vi "_fgv_debug.vi"(7 "Operation":T1=enum."ReadCommand", 8 "error in":errorcluster caption="error in (no error)", 9 "Command in":string, 11 "VISA resource name":refnum<visa-resource-name>) -> (0 "error out":errorcluster, 3 "VISA resource name out":refnum<visa-resource-name>)   [LabVIEW 2020, in "Rohde&Schwarz RTx Oscilloscopes.lvlib" / "rsidr_core.lvlib"]
uses:
  rsidr_core.lvlib
  _type_Operation_Fgv_Debug.ctl
  type_Error_Codes.ctl
  Match Regular Expression.xnode
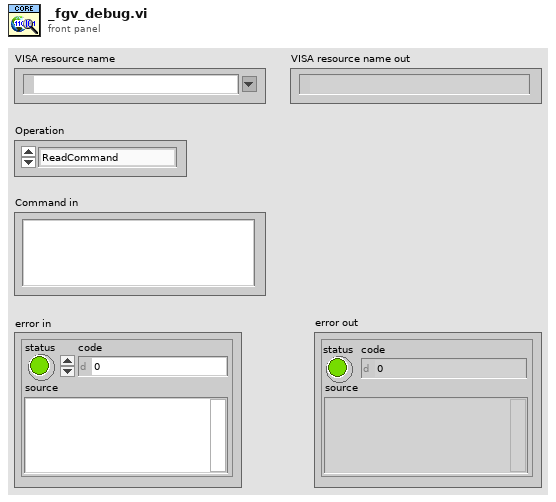
[diagram p1: front panel]
types:
  T1 = typedef "Rohde&Schwarz RTx Oscilloscopes.lvlib/rsidr_core.lvlib/_type_Operation_Fgv_Debug.ctl" = enum16{"Reset", "ReadCommand", "SetCommand"}
  T2 = typedef "Rohde&Schwarz RTx Oscilloscopes.lvlib/rsidr_core.lvlib/type_Error_Codes.ctl" = enum16{"No_error", "VISA_err_ResourceNotFound", "VISA_err_Timeout", "VISA_warn_MoreDataAvailable", "RS_err_MissingCallback", "RS_err_InvalidAttribute", "RS_err_InvalidValue", "RS_err_UnknownResource", "RS_err_AlreadyInitialized", "RS_err_InstrumentStatus", "RS_err_BadRepCapName", "RS_err_TypesMismatch", "RS_err_ValueNotSupported", "RS_err_InvalidRngTable", "RS_err_IDqueryFail", "RS_err_UnexpResponse", "VISA_warn_ConfigNotLoaded", "RS_err_AttributeNotReadable", "RS_err_AttributeNotWritable", "RS_err_InstrumentType", "RS_err_InstrumentOption", "VISA_err_InvalidSize", "RS_err_ReliabilityIndicator", "VISA_warn_UnknownStatus", "VISA_warn_TermCharRead", "VISA_err_IO_error", "RS_err_FunctionNotSupported", "VISA_warn_QueueEmpty"}
  T3 = typedef "Rohde&Schwarz RTx Oscilloscopes.lvlib/rsidr_core.lvlib/type_Session_Data.ctl" = cluster{"IDN string":string, "Instrument FW":string, "Instr type":string, "Instr type for err. msg.":string, "Installed Options":string[], "Ignore Error Messages":string, "Logging params":variant, "OPC Timeout":i32, "VISA Timeout":i32, "STB Poll VISA Timeout":i32, "Additional Flags":i32, "Wait Before Read":i32, "Wait Before Write":i32, "Option String Flags":i32, "IO Segment Size":i64, "VISA Access Mode":T4, "Interface Type":T5, "OPC Wait Mode":T6, "Bin Float Number  Format":T7, "Bin Integer Number Format":T8, "Simulate":bool, "VXIcapable":bool, "Duplicate Session":bool, "Add LF to Write":bool, "Logging":bool, "Fast Sweep":bool, "Query Instrument Status":bool, "Check Range":bool, "Check Options":bool, "OPC-sync Attr Writes":bool, "OPC-sync Attr Queries":bool}
  T4 = typedef "Rohde&Schwarz RTx Oscilloscopes.lvlib/rsidr_core.lvlib/type_VisaAccessMode.ctl" = u16
  T5 = typedef "Rohde&Schwarz RTx Oscilloscopes.lvlib/rsidr_core.lvlib/type_InterfaceType.ctl" = enum16{"Unknown", "GPIB", "VXI", "GPIB_VXI", "ASRL", "PXI", "TCPIP", "USB", "SOCKET"}
  T6 = typedef "Rohde&Schwarz RTx Oscilloscopes.lvlib/rsidr_core.lvlib/type_OPC_Wait_Mode.ctl" = enum16{"STBpolling", "STBpollingSlow", "STBpollingSuperSlow", "ServiceRequest", "OPCquery"}
  T7 = typedef "Rohde&Schwarz RTx Oscilloscopes.lvlib/rsidr_core.lvlib/type_Binary_Float_Number_Format.ctl" = enum16{"Float_4_Bytes_Swapped", "Float_4_Bytes", "Double_8_Bytes_Swapped", "Double_8_Bytes"}
  T8 = typedef "Rohde&Schwarz RTx Oscilloscopes.lvlib/rsidr_core.lvlib/type_Binary_Integer_Number_Format.ctl" = enum16{"Int32_4_Bytes_Swapped", "Int32_4 Bytes", "Int16_2_Bytes_Swapped", "Int16_2_Bytes"}
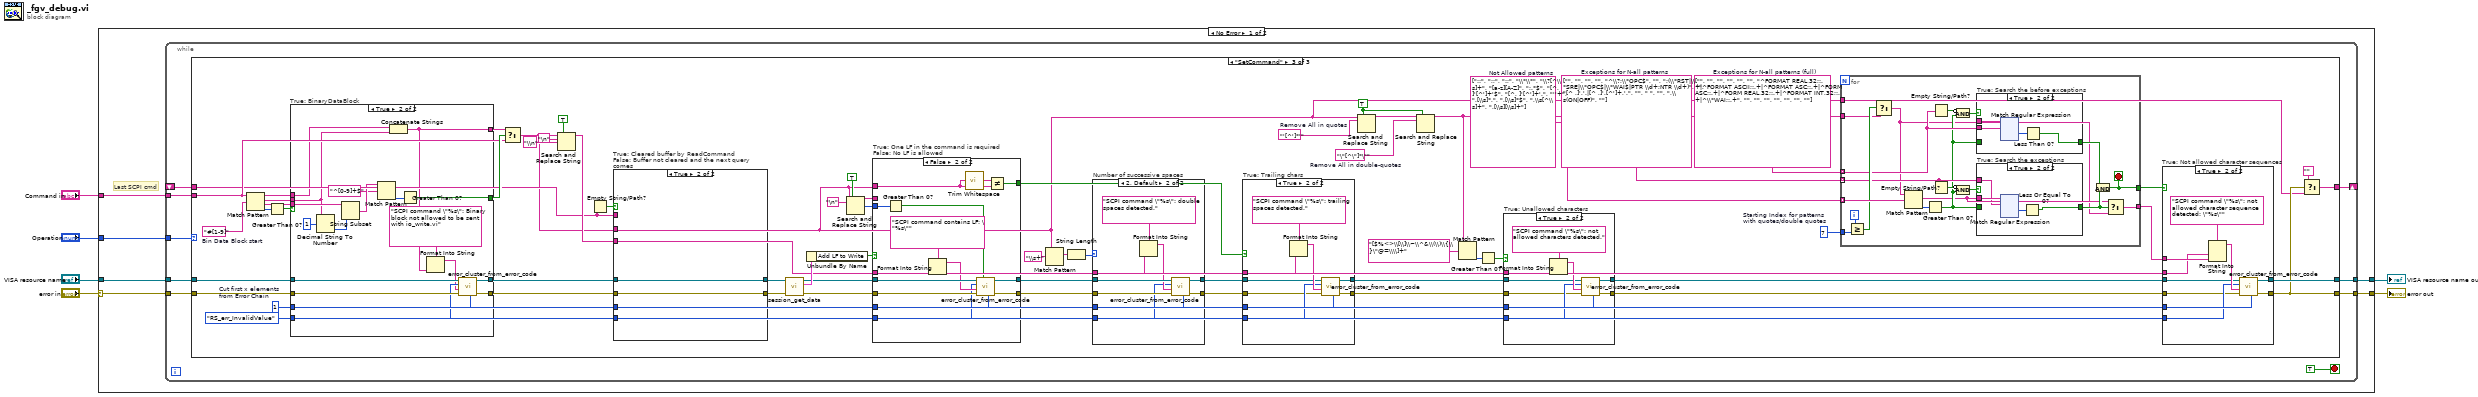
[diagram p0: block diagram]
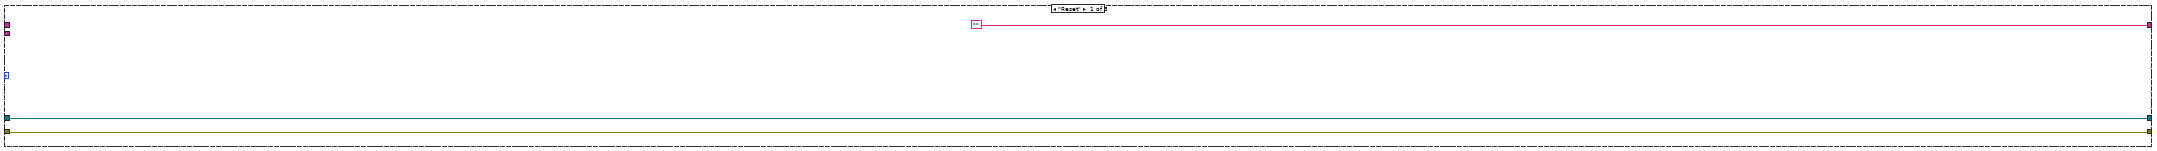
[diagram p2: hidden frame]
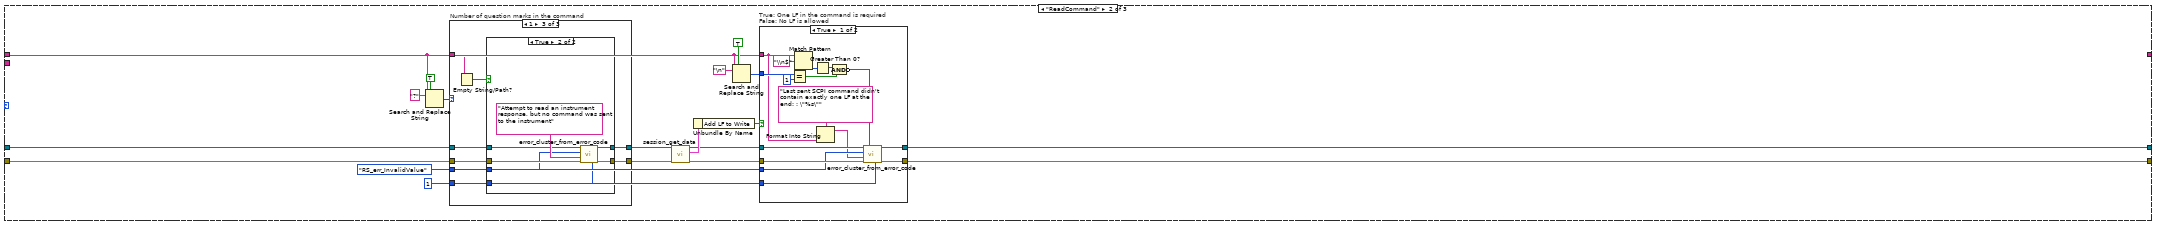
[diagram p3: hidden frame]
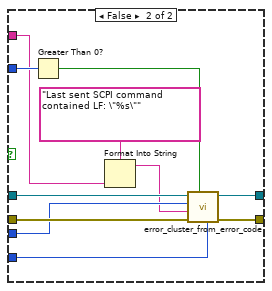
[diagram p4: hidden frame]
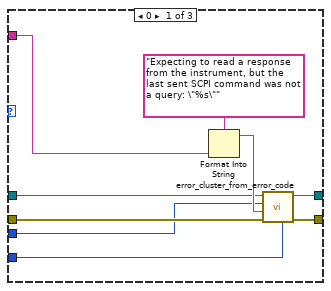
[diagram p5: hidden frame]
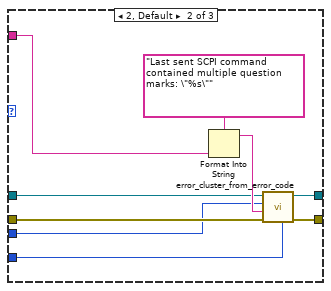
[diagram p6: hidden frame]
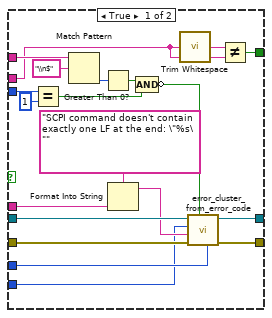
[diagram p14: hidden frame]
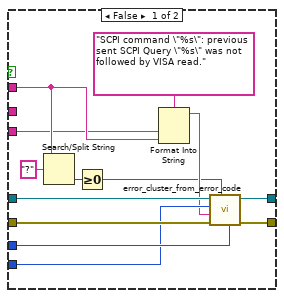
[diagram p16: hidden frame]
diagram:
  n1 = case shown="No Error" "error in" {
    selector: "error in" -> [w8 w536]
    tunnel: [w10 w536] -> w2
    tunnel: "Operation" -> [w12 _]
    tunnel: "Command in" -> [w11 _]
    tunnel: "VISA resource name" -> [w7 w535]
    tunnel: [w9 w535] -> w1
    frame No Error {
      # "Last SCPI cmd"
      n2 = while {
        shift-right: [w18] -> _
        shift-left: _ -> [w17]
        tunnel: w12 -> [w20]
        tunnel: w8 -> [w14]
        tunnel: w11 -> [w19]
        tunnel: w7 -> [w13]
        tunnel: [w16] -> w10
        tunnel: [w15] -> w9
        stop <- TRUE stop-if-true
        n3 = case shown="\"SetCommand\"" w20 {
          tunnel: w19 -> [_ _ w127]
          tunnel: ["" ("Empty String Constant") _ w162] -> w18
          tunnel: w17 -> [_ w28 w126]
          tunnel: w14 -> [w23 w40 w112]
          tunnel: w13 -> [w22 w39 w111]
          tunnel: [w23 w27 w141] -> w16
          tunnel: [w22 w26 w142] -> w15
          frame "Reset" {
          }
          frame "ReadCommand" {
            w25 = 1 ("Cut first x elements\nfrom Error Chain (0)")
            w31 = type_Error_Codes."RS_err_InvalidValue" ("Error Enum in")
            n4 = Search and Replace String(replace all?=TRUE ("replace all? (F)"), input string=w28, search string="?") -> (number of replacements=w41:i32)  [unwired: 5 in, 3 out]
            n5 = case "Number of question marks in the command" shown="1" w41 {
              tunnel: w40 -> [w78 w87 w94]
              tunnel: [w77 w86 w92] -> w38
              tunnel: w28 -> [w76 w85 w96]
              tunnel: w39 -> [w74 w82 w93]
              tunnel: [w73 w84 w91] -> w37
              tunnel: w31 -> [w72 w81 w90]
              tunnel: w25 -> [w71 w80 w89]
              frame 0 {
                n6 = Format Into String(format string="Expecting to read a response from the instrument, but the last sent SCPI command was not a query: \"%s\"", w76) -> (resulting string=w75:string)  [unwired: 2 in, 1 out]
                n7 = call "error_cluster_from_error_code.vi"("Cut first x elements\nfrom Error Chain (0)"=w71, "error in"=w78, "Error Message (\"\")"=w75, "Error Enum in"=w72, "VISA resource name"=w74) -> ("error out"=w77:errorcluster, "VISA resource name out"=w73:refnum<visa-resource-name>)  [unwired: 5 in]
              }
              frame 2, Default {
                n8 = Format Into String(format string="Last sent SCPI command contained multiple question marks: \"%s\"", w85) -> (resulting string=w83:string)  [unwired: 2 in, 1 out]
                n9 = call "error_cluster_from_error_code.vi"("Cut first x elements\nfrom Error Chain (0)"=w80, "error in"=w87, "Error Message (\"\")"=w83, "Error Enum in"=w81, "VISA resource name"=w82) -> ("error out"=w86:errorcluster, "VISA resource name out"=w84:refnum<visa-resource-name>)  [unwired: 5 in]
              }
              frame 1 {
                n10 = Empty String/Path?(string/path=w96) -> (empty?=w95:bool)
                n11 = case shown="True" w95 {
                  tunnel: w94 -> [w98 w104]
                  tunnel: [w98 w102] -> w92
                  tunnel: w93 -> [w97 w103]
                  tunnel: [w97 w101] -> w91
                  tunnel: w90 -> [_ w100]
                  tunnel: w89 -> [_ w99]
                  frame False {
                  }
                  frame True {
                    n12 = call "error_cluster_from_error_code.vi"("Cut first x elements\nfrom Error Chain (0)"=w99, "error in"=w104, "Error Message (\"\")"="Attempt to read an instrument response, but no command was sent to the instrument" ("error message (\"\")"), "Error Enum in"=w100, "VISA resource name"=w103) -> ("error out"=w102:errorcluster, "VISA resource name out"=w101:refnum<visa-resource-name>)  [unwired: 5 in]
                  }
                }
              }
            }
            n13 = call "session_get_data.vi"("error in"=w38, "VISA resource name"=w37) -> ("error out"=w33:errorcluster, "Session User Data out"=w34:T3, "VISA resource name out"=w32:refnum<visa-resource-name>)  [unwired: 6 in, 1 out]
            n14 = Unbundle By Name(w34) -> ("Add LF to Write"=w30:bool)
            n15 = Search and Replace String(replace all?=TRUE ("replace all? (F)"), input string=w28, search string="\n" ("Line Feed Constant")) -> (number of replacements=w29:i32)  [unwired: 5 in, 3 out]
            n16 = case "True: One LF in the command is required\nFalse: No LF is allowed" shown="True" w30 {
              tunnel: w33 -> [w59 w70]
              tunnel: w32 -> [w58 w69]
              tunnel: w31 -> [w57 w68]
              tunnel: w29 -> [w56 w65]
              tunnel: w28 -> [w46 w61]
              tunnel: [w49 w67] -> w27
              tunnel: [w48 w66] -> w26
              tunnel: w25 -> [w44 w60]
              frame True {
                n17 = Equal?(x=w56, y=1) -> (x = y?=w51:bool)
                n18 = Match Pattern(string=w46, regular expression="\\n$") -> (offset past match=w53:i32)  [unwired: 1 in, 3 out]
                n19 = Greater Than 0?(x=w53) -> (x > 0?=w52:bool)
                n20 = Format Into String(format string="Last sent SCPI command didn't contain exactly one LF at the end: : \"%s\"", w46) -> (resulting string=w45:string)  [unwired: 2 in, 1 out]
                n21 = Compound Arithmetic op=AND(w52, w51) -> (invert w50:bool)
                n22 = call "error_cluster_from_error_code.vi"("Cut first x elements\nfrom Error Chain (0)"=w44, "Error Creation Enabled (True)"=w50, "error in"=w59, "Error Message (\"\")"=w45, "Error Enum in"=w57, "VISA resource name"=w58) -> ("error out"=w49:errorcluster, "VISA resource name out"=w48:refnum<visa-resource-name>)  [unwired: 4 in]
              }
              frame False {
                n23 = Greater Than 0?(x=w65) -> (x > 0?=w64:bool)
                n24 = Format Into String(format string="Last sent SCPI command contained LF: \"%s\"", w61) -> (resulting string=w62:string)  [unwired: 2 in, 1 out]
                n25 = call "error_cluster_from_error_code.vi"("Cut first x elements\nfrom Error Chain (0)"=w60, "Error Creation Enabled (True)"=w64, "error in"=w70, "Error Message (\"\")"=w62, "Error Enum in"=w68, "VISA resource name"=w69) -> ("error out"=w67:errorcluster, "VISA resource name out"=w66:refnum<visa-resource-name>)  [unwired: 4 in]
              }
            }
          }
          frame "SetCommand" {
            w106 = string[] ["", "", "", "", "", "", "^FORMAT REAL,32;:.+|^FORMAT ASCII;:.+|^FORMAT ASC;:.+|^FORM ASC;:.+|^FORM REAL,32;:.+|^FORMAT INT,32;:.+|^\\*WAI;:.+", "", "", "", "", "", "", ""]  # Exceptions for N-all patterns (full)
            w118 = 7  # Starting Index for patterns with quotes/double quotes
            w122 = "\"[^\"]*\""  # Remove All in double-quotes
            w114 = "#[1-9]"  # Bin Data Block start
            w132 = string[] ["", "", "", "", "^\\?;\\*OPC$", "", ";(\\*RST|\\*SRE|\\*OPC$|\\*WAI$|PTR \\d+;NTR \\d+)", "", "[^ ,]','.|[^ ,]',[^']+,'.", "", " ", "", ",\\s(ON|OFF)", ""]  # Exceptions for N-all patterns
            w123 = TRUE ("replace all? (F)")
            w107 = "'[^']*'"  # Remove All in quotes
            w146 = string[] ["::", ";;", ":;", "\\*\\*", "\\?[^\\s]+", "[a-z][A-Z]", ";.*$", "[^, ]'[^']+'$", "[^, ]'[^']+'.", "''+", ",[\\s]*,", ",[\\s]*$", ",\\s[^\\s]+", ",[\\s][\\s]+"]  # Not Allowed patterns
            w113 = 1  # Cut first x elements from Error Chain
            w108 = type_Error_Codes."RS_err_InvalidValue" ("Error Enum in")
            n26 = Match Pattern(string=w127, regular expression=w114) -> (before substring=w115:string, match substring=w117:string, after substring=w129:string, offset past match=w131:i32)  [unwired: 1 in]
            n27 = Greater Than 0?(x=w131) -> (x > 0?=w130:bool)
            n28 = case "True: BinaryDataBlock" shown="True" w130 {
              selector: w130 -> [w170 _]
              tunnel: w129 -> [_ w187]
              tunnel: w117 -> [_ w180]
              tunnel: [w170 w182] -> w128
              tunnel: [_ w171] -> w116
              tunnel: w115 -> [_ w181]
              tunnel: w113 -> [_ w175]
              tunnel: w112 -> [w168 w179]
              tunnel: w111 -> [w169 w178]
              tunnel: [w168 w177] -> w110
              tunnel: [w169 w176] -> w109
              tunnel: w108 -> [_ w174]
              frame False {
              }
              frame True {
                n29 = Decimal String To Number(string=w180, offset=1) -> (number=w186:i32)  [unwired: 1 in, 1 out]
                n30 = String Subset(string=w187, length (rest)=w186) -> (substring=w185:string)  [unwired: 1 in]
                n31 = Match Pattern(string=w185, regular expression="^[0-9]+$") -> (offset past match=w183:i32)  [unwired: 1 in, 3 out]
                n32 = Concatenate Strings(w181, w180) -> (w171:string)
                n33 = Greater Than 0?(x=w183) -> (x > 0?=w182:bool)
                n34 = Format Into String(format string="SCPI command \"%s\": Binary block not allowed to be sent with io_write.vi", w171) -> (resulting string=w172:string)  [unwired: 2 in, 1 out]
                n35 = call "error_cluster_from_error_code.vi"("Cut first x elements\nfrom Error Chain (0)"=w175, "error in"=w179, "Error Message (\"\")"=w172, "Error Enum in"=w174, "VISA resource name"=w178) -> ("error out"=w177:errorcluster, "VISA resource name out"=w176:refnum<visa-resource-name>)  [unwired: 5 in]
              }
            }
            n36 = Select(t=w116, s=w128, f=w127) -> (s? t:f=w119:string)
            n37 = Search and Replace String(replace all?=TRUE ("replace all? (F)"), input string=w119, search string="\n" ("Line Feed Constant"), replace string="\\n" ("input string")) -> (result string=w133:string)  [unwired: 4 in, 3 out]
            n38 = Empty String/Path?(string/path=w126) -> (empty?=w163:bool)
            n39 = case "True: Cleared buffer by ReadCommand\nFalse: Buffer not cleared and the next query comes" shown="True" w163 {
              tunnel: w126 -> [w527 _]
              tunnel: w110 -> [w531 w534]
              tunnel: [w530 w534] -> w153
              tunnel: w119 -> [_ _]
              tunnel: w113 -> [w526 _]
              tunnel: w108 -> [w525 _]
              tunnel: w109 -> [w524 w533]
              tunnel: [w523 w533] -> w154
              tunnel: w133 -> [w520 _]
              frame False {
                n40 = Search/Split String(string=w527, search string/char (-)="?") -> (offset of match=w529:i32)  [unwired: 1 in, 2 out]
                n41 = Greater Or Equal To 0?(x=w529) -> (x >= 0?=w521:bool)
                n42 = Format Into String(format string="SCPI command \"%s\": previous sent SCPI Query \"%s\" was not followed by VISA read.", w520, w527) -> (resulting string=w522:string)  [unwired: 2 in, 1 out]
                n43 = call "error_cluster_from_error_code.vi"("Cut first x elements\nfrom Error Chain (0)"=w526, "Error Creation Enabled (True)"=w521, "error in"=w531, "Error Message (\"\")"=w522, "Error Enum in"=w525, "VISA resource name"=w524) -> ("error out"=w530:errorcluster, "VISA resource name out"=w523:refnum<visa-resource-name>)  [unwired: 4 in]
              }
              frame True {
              }
            }
            n44 = call "session_get_data.vi"("error in"=w153, "VISA resource name"=w154) -> ("error out"=w158:errorcluster, "Session User Data out"=w159:T3, "VISA resource name out"=w157:refnum<visa-resource-name>)  [unwired: 6 in, 1 out]
            n45 = Unbundle By Name(w159) -> ("Add LF to Write"=w156:bool)
            n46 = Search and Replace String(replace all?=TRUE ("replace all? (F)"), input string=w119, search string="\n" ("Line Feed Constant")) -> (result string=w121:string, number of replacements=w155:i32)  [unwired: 5 in, 2 out]
            n47 = case "True: One LF in the command is required\nFalse: No LF is allowed" shown="False" w156 {
              tunnel: w158 -> [w494 w508]
              tunnel: w157 -> [w493 w507]
              tunnel: w155 -> [w492 w504]
              tunnel: w119 -> [w482 w496]
              tunnel: [w485 w506] -> w151
              tunnel: [w484 w505] -> w152
              tunnel: w113 -> [w480 w500]
              tunnel: w108 -> [w479 w499]
              tunnel: w133 -> [w478 w498]
              tunnel: w121 -> [w476 _]
              tunnel: [w475 w495] -> w120
              frame True {
                n48 = Equal?(x=w492, y=1) -> (x = y?=w487:bool)
                n49 = Match Pattern(string=w482, regular expression="\\n$") -> (offset past match=w489:i32)  [unwired: 1 in, 3 out]
                n50 = Greater Than 0?(x=w489) -> (x > 0?=w488:bool)
                n51 = Format Into String(format string="SCPI command doesn't contain exactly one LF at the end: \"%s\"", w478) -> (resulting string=w481:string)  [unwired: 2 in, 1 out]
                n52 = Compound Arithmetic op=AND(w488, w487) -> (invert w486:bool)
                n53 = call "Trim Whitespace.vi"("string"=w476) -> ("trimmed string"=w477:string)  [unwired: 1 in]
                n54 = call "error_cluster_from_error_code.vi"("Cut first x elements\nfrom Error Chain (0)"=w480, "Error Creation Enabled (True)"=w486, "error in"=w494, "Error Message (\"\")"=w481, "Error Enum in"=w479, "VISA resource name"=w493) -> ("error out"=w485:errorcluster, "VISA resource name out"=w484:refnum<visa-resource-name>)  [unwired: 4 in]
                n55 = Not Equal?(x=w477, y=w476) -> (x != y?=w475:bool)
              }
              frame False {
                n56 = Greater Than 0?(x=w504) -> (x > 0?=w503:bool)
                n57 = Format Into String(format string="SCPI command contains LF: \"%s\"", w498) -> (resulting string=w501:string)  [unwired: 2 in, 1 out]
                n58 = call "Trim Whitespace.vi"("string"=w496) -> ("trimmed string"=w497:string)  [unwired: 1 in]
                n59 = call "error_cluster_from_error_code.vi"("Cut first x elements\nfrom Error Chain (0)"=w500, "Error Creation Enabled (True)"=w503, "error in"=w508, "Error Message (\"\")"=w501, "Error Enum in"=w499, "VISA resource name"=w507) -> ("error out"=w506:errorcluster, "VISA resource name out"=w505:refnum<visa-resource-name>)  [unwired: 4 in]
                n60 = Not Equal?(x=w497, y=w496) -> (x != y?=w495:bool)
              }
            }
            n61 = Match Pattern(string=w119, regular expression="\\s+") -> (match substring=w166:string)  [unwired: 1 in, 3 out]
            n62 = String Length(string=w166) -> (length=w167:i32)
            n63 = case "Number of successive spaces" shown="2, Default" w167 {
              tunnel: w151 -> [w510 w519]
              tunnel: [w510 w518] -> w140
              tunnel: w152 -> [w509 w516]
              tunnel: [w509 w515] -> w139
              tunnel: w113 -> [_ w513]
              tunnel: w108 -> [_ w512]
              tunnel: w133 -> [_ w511]
              frame 0, 1 {
              }
              frame 2, Default {
                n64 = Format Into String(format string="SCPI command \"%s\": double spaces detected.", w511) -> (resulting string=w514:string)  [unwired: 2 in, 1 out]
                n65 = call "error_cluster_from_error_code.vi"("Cut first x elements\nfrom Error Chain (0)"=w513, "error in"=w519, "Error Message (\"\")"=w514, "Error Enum in"=w512, "VISA resource name"=w516) -> ("error out"=w518:errorcluster, "VISA resource name out"=w515:refnum<visa-resource-name>)  [unwired: 5 in]
              }
            }
            n66 = case "True: Trailing chars" shown="True" w120 {
              tunnel: w140 -> [w190 w195]
              tunnel: [w190 w193] -> w138
              tunnel: w139 -> [w189 w194]
              tunnel: [w189 w192] -> w137
              tunnel: w113 -> [_ w197]
              tunnel: w108 -> [_ w196]
              tunnel: w133 -> [_ w191]
              frame False {
              }
              frame True {
                n67 = Format Into String(format string="SCPI command \"%s\": trailing spaces detected.", w191) -> (resulting string=w198:string)  [unwired: 2 in, 1 out]
                n68 = call "error_cluster_from_error_code.vi"("Cut first x elements\nfrom Error Chain (0)"=w197, "error in"=w195, "Error Message (\"\")"=w198, "Error Enum in"=w196, "VISA resource name"=w194) -> ("error out"=w193:errorcluster, "VISA resource name out"=w192:refnum<visa-resource-name>)  [unwired: 5 in]
              }
            }
            n69 = Search and Replace String(replace all?=w123, input string=w119, search string=w107) -> (result string=w124:string)  [unwired: 5 in, 3 out]
            n70 = Search and Replace String(replace all?=w123, input string=w124, search string=w122) -> (result string=w125:string)  [unwired: 5 in, 3 out]
            n71 = Match Pattern(string=w125, regular expression="[$%<>\\[\\]\\~\\^&\\(\\)\\{\\}\"@=\\\\]+") -> (offset past match=w148:i32)  [unwired: 1 in, 3 out]
            n72 = Greater Than 0?(x=w148) -> (x > 0?=w149:bool)
            n73 = case "True: Unallowed characters" shown="True" w149 {
              tunnel: w138 -> [w465 w470]
              tunnel: [w465 w468] -> w143
              tunnel: w137 -> [w464 w469]
              tunnel: [w464 w467] -> w147
              tunnel: w113 -> [_ w472]
              tunnel: w108 -> [_ w471]
              tunnel: w133 -> [_ w466]
              frame False {
              }
              frame True {
                n74 = Format Into String(format string="SCPI command \"%s\": not allowed characters detected.", w466) -> (resulting string=w473:string)  [unwired: 2 in, 1 out]
                n75 = call "error_cluster_from_error_code.vi"("Cut first x elements\nfrom Error Chain (0)"=w472, "error in"=w470, "Error Message (\"\")"=w473, "Error Enum in"=w471, "VISA resource name"=w469) -> ("error out"=w468:errorcluster, "VISA resource name out"=w467:refnum<visa-resource-name>)  [unwired: 5 in]
              }
            }
            n76 = for {
              tunnel: w146 -> [w219] mode=indexing
              tunnel: [w205] -> w145
              tunnel: [w202] -> w144
              tunnel: w125 -> [w212]
              tunnel: w132 -> [w210] mode=indexing
              tunnel: w119 -> [w215]
              tunnel: w118 -> [w211]
              tunnel: w106 -> [w207] mode=indexing
              i -> [w214]
              stop <- w205 stop-if-true
              n77 = Greater Or Equal?(x=w214, y=w211) -> (x >= y?=w213:bool)
              n78 = Select(t=w215, s=w213, f=w212) -> (s? t:f=w200:string)
              n79 = Match Pattern(string=w200, regular expression=w219) -> (match substring=w201:string, offset past match=w218:i32)  [unwired: 1 in, 2 out]
              n80 = Greater Than 0?(x=w218) -> (x > 0?=w206:bool)
              n81 = Empty String/Path?(string/path=w207) -> (empty?=w209:bool)
              n82 = Empty String/Path?(string/path=w210) -> (empty?=w217:bool)
              n83 = Compound Arithmetic op=AND(invert w209, w206) -> (w208:bool)
              n84 = Compound Arithmetic op=AND(invert w217, w206) -> (w216:bool)
              n85 = case "True: Search the before exceptions" shown="True" w208 {
                tunnel: w206 -> [w220 _]
                tunnel: w200 -> [_ w224]
                tunnel: w207 -> [_ w223]
                tunnel: [w220 w221] -> w204
                frame False {
                }
                frame True {
                  n86 = xnode ("Match Regular Expression")("input string"=w224, "regular expression"=w223) -> ("offset past match"=w222:i32)  [unwired: 4 in, 4 out]
                  n87 = Less Than 0?(x=w222) -> (x < 0?=w221:bool)
                }
              }
              n88 = case "True: Search the exceptions" shown="True" w216 {
                tunnel: w206 -> [w336 _]
                tunnel: w201 -> [_ w340]
                tunnel: w210 -> [_ w339]
                tunnel: [w336 w337] -> w203
                frame False {
                }
                frame True {
                  n89 = xnode ("Match Regular Expression")("input string"=w340, "regular expression"=w339) -> ("offset past match"=w338:i32)  [unwired: 4 in, 4 out]
                  n90 = Less Or Equal To 0?(x=w338) -> (x <= 0?=w337:bool)
                }
              }
              n91 = And(x=w204, y=w203) -> (x .and. y?=w205:bool)
              n92 = Select(t=w201, s=w203, f=w200) -> (s? t:f=w202:string)
            }
            n93 = case "True: Not allowed character sequences" shown="True" w145 {
              tunnel: w143 -> [w453 w459]
              tunnel: [w453 w457] -> w141
              tunnel: w147 -> [w452 w458]
              tunnel: [w452 w456] -> w142
              tunnel: w113 -> [_ w461]
              tunnel: w108 -> [_ w460]
              tunnel: w144 -> [_ w455]
              tunnel: w133 -> [_ w454]
              frame False {
              }
              frame True {
                n94 = Format Into String(format string="SCPI command \"%s\": not allowed character sequence detected: \"%s\"", w454, w455) -> (resulting string=w462:string)  [unwired: 2 in, 1 out]
                n95 = call "error_cluster_from_error_code.vi"("Cut first x elements\nfrom Error Chain (0)"=w461, "error in"=w459, "Error Message (\"\")"=w462, "Error Enum in"=w460, "VISA resource name"=w458) -> ("error out"=w457:errorcluster, "VISA resource name out"=w456:refnum<visa-resource-name>)  [unwired: 5 in]
              }
            }
            n96 = Select(t="" ("Empty String Constant"), s=w141, f=w119) -> (s? t:f=w162:string)
          }
        }
      }
    }
    frame Error {
    }
  }
  "error out" <- w2
  "VISA resource name out" <- w1
